vi "Sweep Table Filename (Read).vi"(6 "ISOBUS address":T5=-1 caption="ISOBUS address (-1)", 8 "error in":errorcluster, 11 "Mercury Reference In":T2) -> (0 "error out":errorcluster, 2 "Sweep Table Filename":string, 3 "Mercury Reference Out":T2, 4 "Valid?":T1)   [LabVIEW 2015, in "Mercury iXX.lvlib" / "Control Loop.lvlib"]
doc: "Read the filename of the sweep table."
uses:
  Control Loop.lvlib
  Controls/Mercury Reference.ctl
  Controls/Comms Transport Layer.ctl
  Private/Controls/Query Dynamic Reference.ctl
  Controls/ISOBus Address.ctl
  Controls/Is Valid LED.ctl
  Private/Controls/Command Verbs.ctl
  Mercury iXX.lvlib
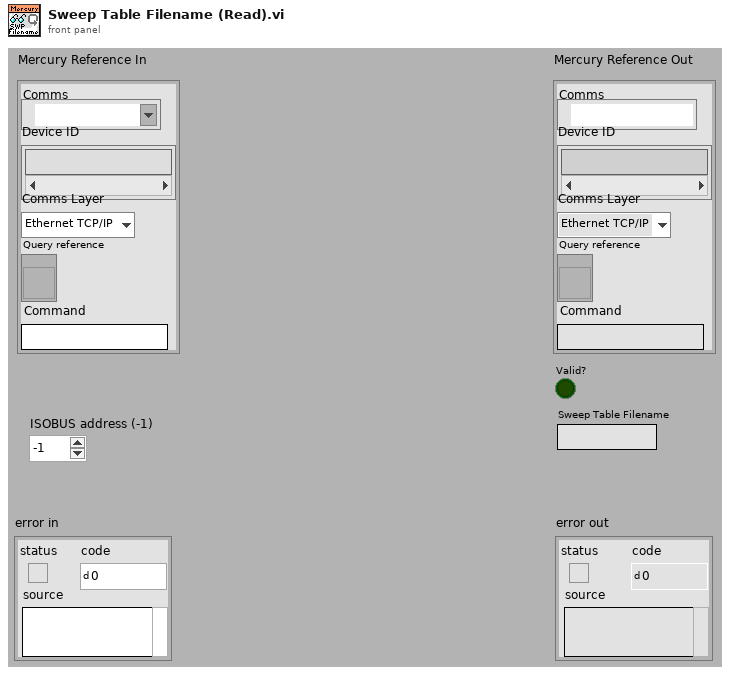
[diagram p1: front panel]
types:
  T1 = typedef "Mercury iXX.lvlib/Is Valid LED.ctl" = bool
  T2 = typedef "Mercury iXX.lvlib/Mercury Reference.ctl" = cluster{"Comms":refnum<visa-resource-name>, "Device ID":string[], "Comms Layer":T3, "Command":string, "Query reference":T4}
  T3 = typedef "Mercury iXX.lvlib/Comms Transport Layer.ctl" = enum16{"Ethernet TCP/IP", "USB", "ISOBus - RS-232", "GPIB"}
  T4 = typedef "Mercury iXX.lvlib/Query Dynamic Reference.ctl" = refnum<vi>
  T5 = typedef "Mercury iXX.lvlib/ISOBus Address.ctl" = i32
  T6 = typedef "Mercury iXX.lvlib/Command Verbs.ctl" = string
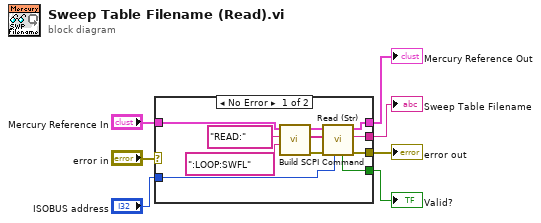
[diagram p0: block diagram]
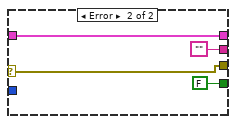
[diagram p2: hidden frame]
diagram:
  n1 = case shown="No Error" "error in" {
    selector: "error in" -> [_ w21]
    tunnel: "Mercury Reference In" -> [w13 w22]
    tunnel: [w12 w22] -> w1
    tunnel: [w9 w21] -> w4
    tunnel: "ISOBUS address" -> [w8 _]
    tunnel: [w11 ""] -> w2
    tunnel: [w10 FALSE ("Valid?")] -> w3
    frame No Error {
      n2 = call "Build SCPI Command.vi"("Noun(s)"=":LOOP:SWFL" ("Command"), "Verb"=T6 "READ:", "Mercury Reference In"=w13) -> ("error out"=w14:errorcluster, "SCPI Message(s)"=w17:string[], "Mercury Reference Out"=w16:T2)  [unwired: 1 in, 5 out]
      n3 = call "Read (Str).vi"("ISOBUS address"=w8, "error in"=w14, "SCPI Message(s)"=w17, "Mercury Reference In"=w16) -> ("error out"=w9:errorcluster, "Response"=w11:string, "Mercury Reference Out"=w12:T2, "Valid?"=w10:T1)  [unwired: 4 out]
    }
    frame Error {
    }
  }
  "Mercury Reference Out" <- w1
  "Sweep Table Filename" <- w2
  "error out" <- w4
  "Valid?" <- w3
